vi "Zmienna Globalna 03.vi"() -> ()   [LabVIEW 2020]
uses:
  Zmienna Globalna.vi
panel:
  out "Waveform Chart":dbl(graph)
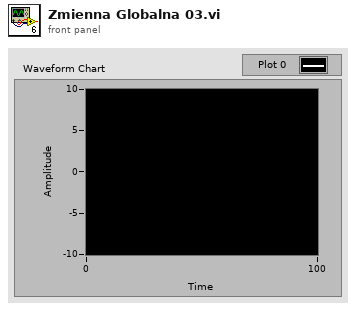
[diagram p1: front panel]
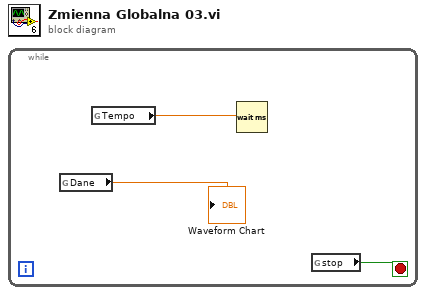
[diagram p0: block diagram]
diagram:
  n1 = while {
    stop <- w3 stop-if-true
    n2 = global read "Zmienna Globalna.vi" "Dane"() -> (→"Waveform Chart":dbl)
    n3 = global read "Zmienna Globalna.vi" "Tempo"() -> (w1:dbl)
    n4 = Wait (ms)(milliseconds to wait=w1) -> ()  [unwired: 1 out]
    n5 = global read "Zmienna Globalna.vi" "stop"() -> (w3:bool)
  }
